vi "Get Current Position TP.vi"(8 "error in (no error)":errorcluster caption="entrée d'erreur (pas d'erreur)", 10 "controllerAddress":i32, 11 "SMC100 in":refnum<k24>) -> (0 "error out":errorcluster caption="sortie d'erreur", 1 "controllerState":string, 2 "CurrentPosition":dbl, 3 "SMC100 out":refnum<k24>)   [LabVIEW 2024, in "SMC100.lvlib"]
uses:
  SMC100.lvlib
  Newport.SMC100.CommandInterface
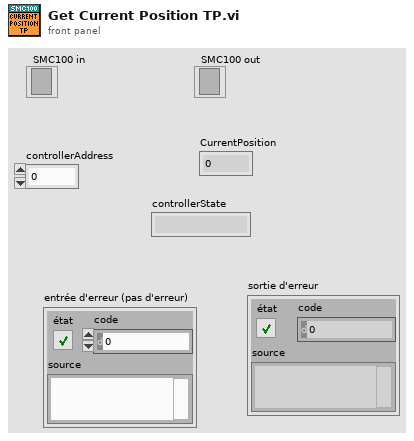
[diagram p1: front panel]
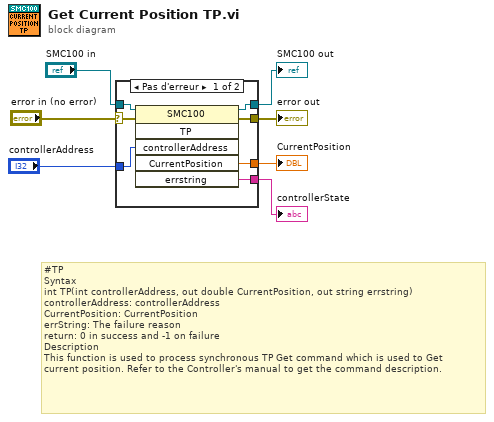
[diagram p0: block diagram]
diagram:
  # "#TP\nSyntax\nint TP(int controllerAddress, out double CurrentPosition, out string errstring)\ncontrollerAddress: controllerAddress\nCurrentPosition: CurrentPosition\nerrString: The failure reason\nreturn: 0 in success and -1 on failure\nDescription\nThis function is used to process synchronous TP Get command which is used to Get\ncurrent position. Refer to the Controller's manual to get the command description."
  n1 = case shown="Pas d'erreur" "error in (no error)" {
    selector: "error in (no error)" -> [w14 w15]
    tunnel: [w13 w15] -> w6
    tunnel: "SMC100 in" -> [w12 w16]
    tunnel: [w11 w16] -> w4
    tunnel: "controllerAddress" -> [w10 _]
    tunnel: [w9 _] -> w2
    tunnel: [w8 _] -> w1
    frame No Error {
      n2 = invoke class="SMC100" method="TP"(reference=w12, error in=w14, "controllerAddress"=w10) -> (reference out=w11:refnum<k24>, error out=w13:errorcluster, "CurrentPosition"=w8:dbl, "errstring"=w9:string)  [unwired: 3 in, 2 out]
    }
    frame Error {
    }
  }
  "error out" <- w6
  "SMC100 out" <- w4
  "controllerState" <- w2
  "CurrentPosition" <- w1
